vi "LO_YTO-count2freq_naoj.vi"(7 "f max":sgl format="%.2f", 8 "f min":sgl format="%.2f", 9 "YTO count":u16) -> (0 "YTO freq.":sgl format="%.2f")   [LabVIEW 2017]
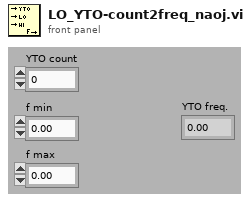
[diagram p1: front panel]
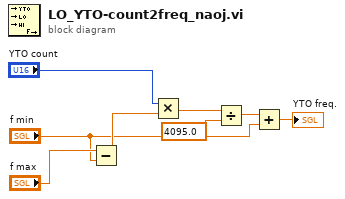
[diagram p0: block diagram]
diagram:
  n1 = Subtract(x="f max", y="f min") -> (x-y=w8:sgl)
  n2 = Multiply(x="YTO count", y=w8) -> (x*y=w6:sgl)
  n3 = Divide(x=w6, y=4095.0) -> (x/y=w3:dbl)
  n4 = Add(x=w3, y="f min") -> (x+y=→"YTO freq.":dbl)
